vi "FTW-CodeGen-Image-Rectangle.vi"(1 "Fill Color":u32(colorbox)=16777216, 2 "Initial Picture":picture, 4 "Rectangle":T1 {"Left" format="%dpx"; "Top" format="%dpx"; "Right" format="%dpx"; "Bottom" format="%dpx"}, 5 "Border Color":u32(colorbox), 8 "Border Width":u8=1 format="%dpx") -> (7 "Picture":picture)   [LabVIEW 2015]
panel:
  # "Inputs"
  # "Outputs"
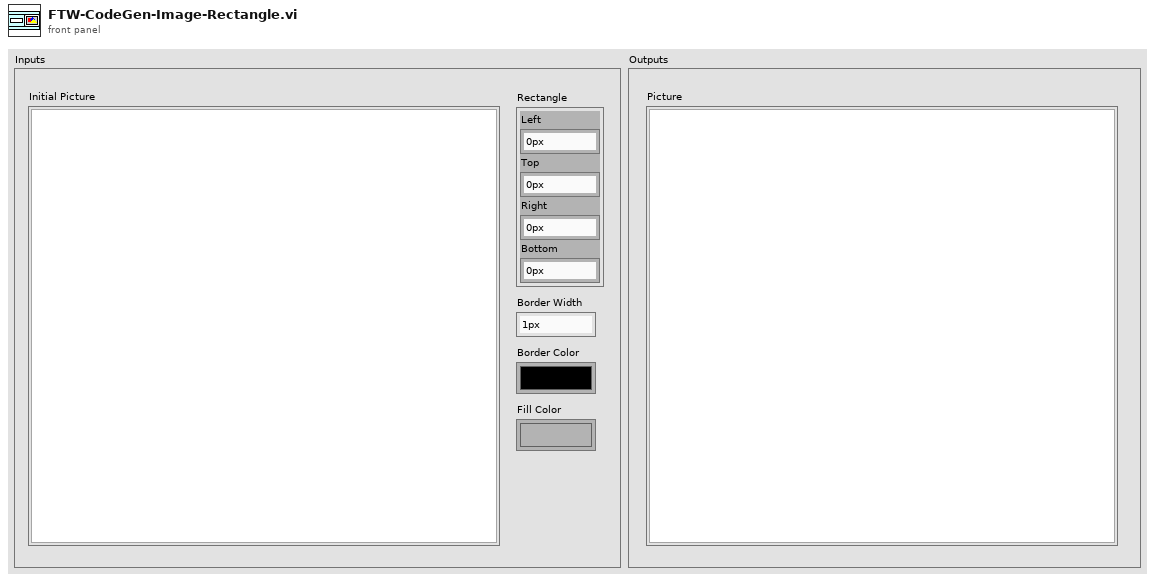
[diagram p1: front panel]
types:
  T1 = cluster{"Left":i32, "Top":i32, "Right":i32, "Bottom":i32}
  T2 = cluster{"Left":i16, "Top":i16, "Right":i16, "Bottom":i16}
  T3 = cluster{"Select Pen Opcode":i16, "Select Pen Size":i32, "PictPen ID":i32, "pen mask":i32, "Border Color":u32, "Border Width":i16, "Style":enum32{"Solid", "Dash", "Dot", "DashDot", "DashDotDot"}, "Frame Rect Opcode":i16, "Frame Rect Size":i32, "top":i16, "left":i16, "bottom":i16, "right":i16}
  T4 = cluster{"Select Pen Opcode":i16, "Select Pen Size":i32, "PictPen ID":i32, "pen mask":i32, "Fill Color":u32, "Border Width (unused)":i16, "Style":enum32{"Solid", "Dash", "Dot", "DashDot", "DashDotDot"}, "Paint Rect Opcode":i16, "Paint Rect Size":i32, "top":i16, "left":i16, "bottom":i16, "right":i16, "Select Pen Opcode 2":i16, "size 2":i32, "PictPen ID 2":i32, "pen mask 2":i32, "Border Color":u32, "Border Width":i16, "Style 2":enum32{"Solid", "Dash", "Dot", "DashDot", "DashDotDot"}, "Frame Rect Opcode":i16, "Frame Rect Size":i32, "top2":i16, "left2":i16, "bottom2":i16, "right2":i16}
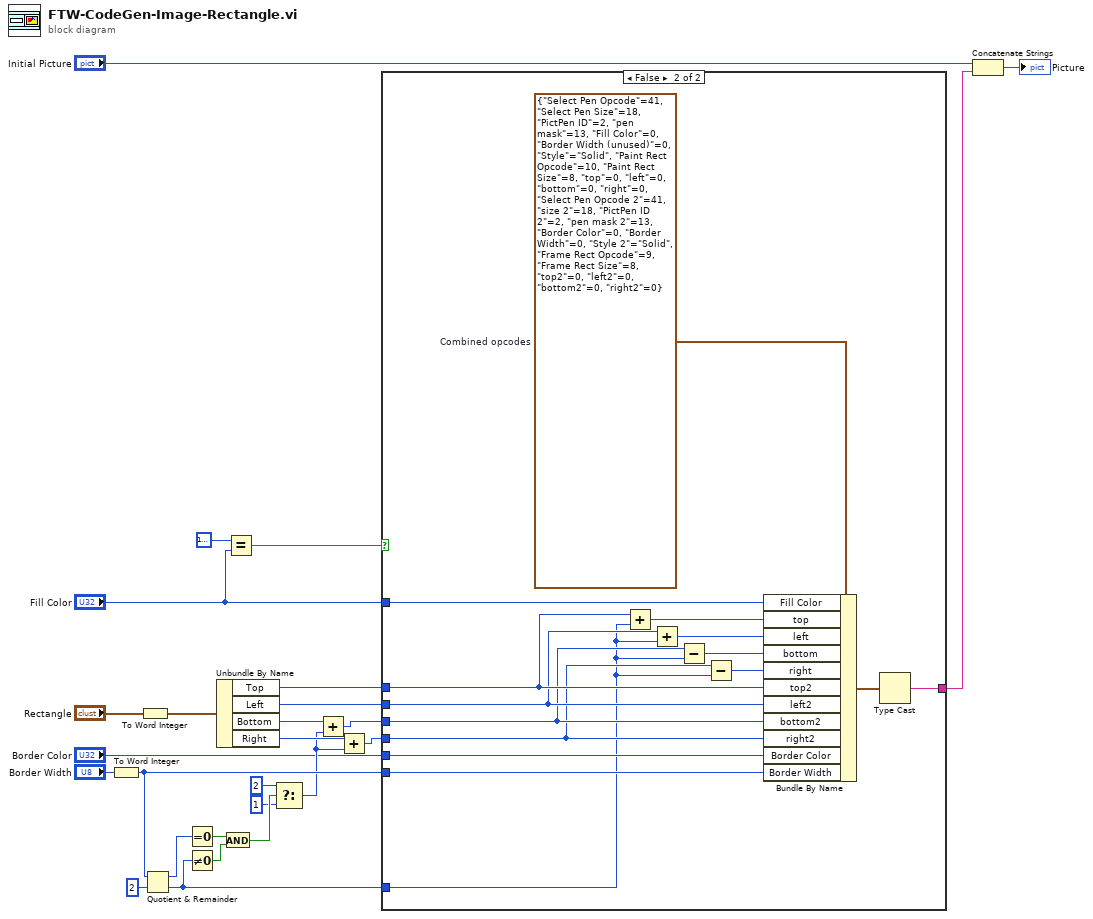
[diagram p0: block diagram]
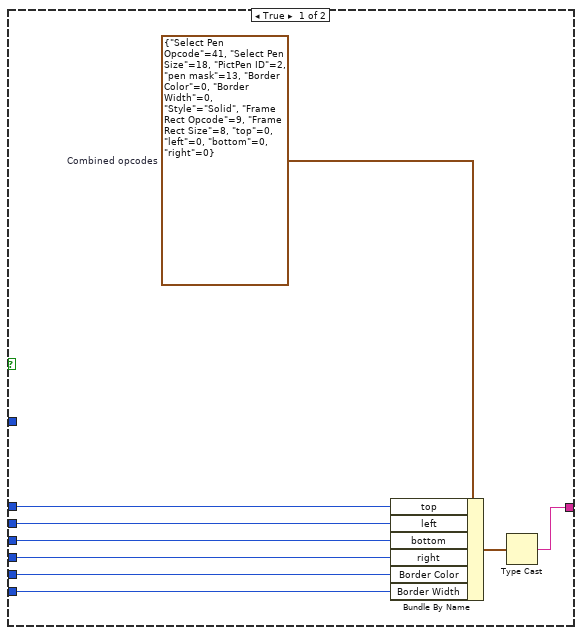
[diagram p2: hidden frame]
diagram:
  n1 = To Word Integer(number="Border Width") -> (16bit integer=w13:i16)
  n2 = To Word Integer(number="Rectangle") -> (16bit integer=w7:T2)
  n3 = Quotient & Remainder(x=w13, y=i16 2) -> (x-y*floor(x/y)=w15:i16, floor(x/y)=w8:i16)
  n4 = Equal To 0?(x=w15) -> (x = 0?=w16:bool)
  n5 = Not Equal To 0?(x=w8) -> (x != 0?=w14:bool)
  n6 = Unbundle By Name(w7) -> ("Top"=w23:i16, "Left"=w22:i16, "Bottom"=w24:i16, "Right"=w25:i16)
  n7 = And(x=w16, y=w14) -> (x .and. y?=w19:bool)
  n8 = Equal?(x=u32 16777216 ("Fill Color"), y="Fill Color") -> (x = y?=w9:bool)
  n9 = Select(t=i16 2, s=w19, f=i16 1) -> (s? t:f=w12:i16)
  n10 = Add(x=w24, y=w12) -> (x+y=w11:i16)
  n11 = Add(x=w25, y=w12) -> (x+y=w10:i16)
  n12 = case shown="False" w9 {
    tunnel: w23 -> [w35 w44]
    tunnel: w22 -> [w34 w42]
    tunnel: "Border Color" -> [w33 w50]
    tunnel: [w32 w49] -> w21
    tunnel: w13 -> [w31 w48]
    tunnel: w11 -> [w29 w40]
    tunnel: w10 -> [w28 w38]
    tunnel: "Fill Color" -> [_ w45]
    tunnel: w8 -> [_ w36]
    frame True {
      w30 = T3 {"Select Pen Opcode"=41, "Select Pen Size"=18, "PictPen ID"=2, "pen mask"=13, "Border Color"=0, "Border Width"=0, "Style"=enum."Solid", "Frame Rect Opcode"=9, "Frame Rect Size"=8, "top"=0, "left"=0, "bottom"=0, "right"=0}  # Combined opcodes
      n13 = Bundle By Name(cluster=w30, "top"=w35, "left"=w34, "bottom"=w29, "right"=w28, "Border Color"=w33, "Border Width"=w31) -> (w27:T3)
      n14 = Type Cast(x=w27) -> (*(type *) &x=w32:string)  [unwired: 1 in]
    }
    frame False {
      w47 = T4 {"Select Pen Opcode"=41, "Select Pen Size"=18, "PictPen ID"=2, "pen mask"=13, "Fill Color"=0, "Border Width (unused)"=0, "Style"=enum."Solid", "Paint Rect Opcode"=10, "Paint Rect Size"=8, "top"=0, "left"=0, "bottom"=0, "right"=0, "Select Pen Opcode 2"=41, "size 2"=18, "PictPen ID 2"=2, "pen mask 2"=13, "Border Color"=0, "Border Width"=0, "Style 2"=enum."Solid", "Frame Rect Opcode"=9, "Frame Rect Size"=8, "top2"=0, "left2"=0, "bottom2"=0, "right2"=0}  # Combined opcodes
      n15 = Add(x=w44, y=w36) -> (x+y=w43:i16)
      n16 = Add(x=w42, y=w36) -> (x+y=w41:i16)
      n17 = Subtract(x=w40, y=w36) -> (x-y=w39:i16)
      n18 = Subtract(x=w38, y=w36) -> (x-y=w37:i16)
      n19 = Bundle By Name(cluster=w47, "Fill Color"=w45, "top"=w43, "left"=w41, "bottom"=w39, "right"=w37, "top2"=w44, "left2"=w42, "bottom2"=w40, "right2"=w38, "Border Color"=w50, "Border Width"=w48) -> (w46:T4)
      n20 = Type Cast(x=w46) -> (*(type *) &x=w49:string)  [unwired: 1 in]
    }
  }
  n21 = Concatenate Strings("Initial Picture", w21) -> (→"Picture":picture)
